vi "Extract Lines on Grass.vi"(8 "error in (no error)":errorcluster, 11 "Image Src":T1) -> (0 "error out":errorcluster, 2 "Number of Particles":i32, 3 "Image Out":T1, 7 "Number of Particles1":i32)   [LabVIEW 2009]
doc: "VI which takes an image and outputs marked regions. One for the left and one for the right"
uses:
  <vilib>/vision/Image Controls.llb/IMAQ Image.ctl
  <vilib>/vision/NI_Vision_Development_Module.lvlib
panel:
  out "Image Dst Out":T1(plugin-control)
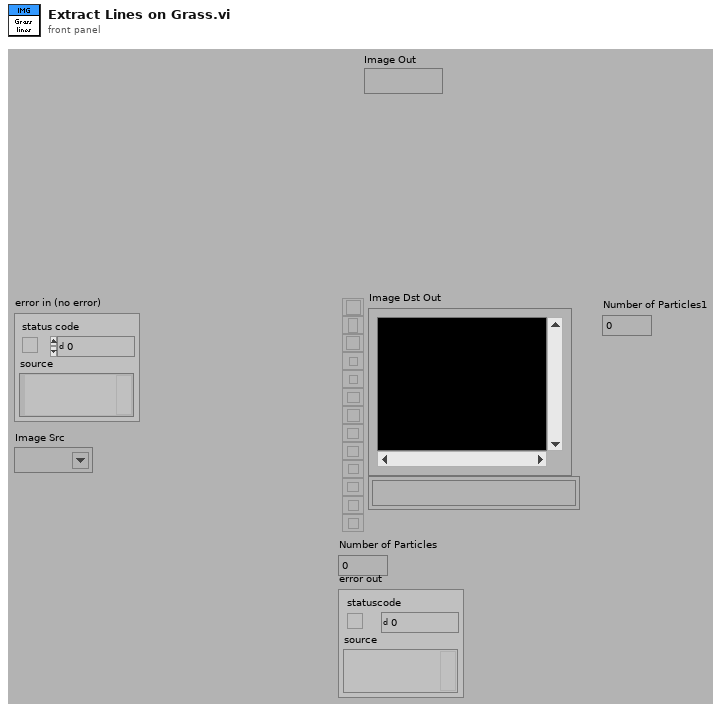
[diagram p1: front panel]
types:
  T1 = typedef "IMAQ Image.ctl" = refnum<image>
  T2 = typedef "Image Type" = u32
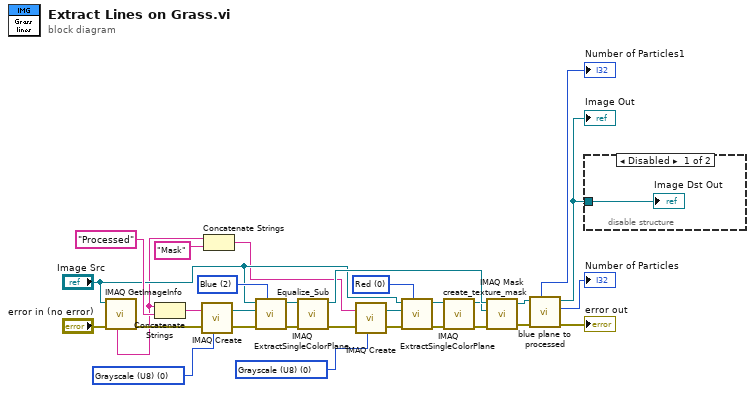
[diagram p0: block diagram]
diagram:
  w18 = T2 0 items=["Grayscale (U8)", "Grayscale (I16)", "Grayscale (SGL)", "Complex (CSG)", "RGB (U32)", "HSL (U32)", "RGB (U64)"] ("Image Type")
  w21 = 0 items=["Red", "Green", "Blue", "Hue", "Saturation", "Luminance", "Value", "Intensity"] ("Color Plane")
  w25 = 2 items=["Red", "Green", "Blue", "Hue", "Saturation", "Luminance", "Value", "Intensity"] ("Color Plane")
  w28 = T2 0 items=["Grayscale (U8)", "Grayscale (I16)", "Grayscale (SGL)", "Complex (CSG)", "RGB (U32)", "HSL (U32)", "RGB (U64)"] ("Image Type")
  n1 = call "IMAQ GetImageInfo"("error in (no error)"="error in (no error)", "Image"="Image Src") -> ("error out"=w10:errorcluster, "Image Name"=w4:string)  [unwired: 8 out]
  n2 = Concatenate Strings(w4, "Processed" ("Image Name")) -> (w6:string)
  n3 = call "IMAQ Create"("Image Name"=w6, "Image Type"=w18, "error in (no error)"=w10) -> ("New Image"=w20:T1, "error out"=w19:errorcluster)  [unwired: 1 in, 1 out]
  n4 = Concatenate Strings(w4, "Mask" ("Image Name")) -> (w7:string)
  n5 = call "IMAQ ExtractSingleColorPlane"("Color Plane"=w25, "error in (no error)"=w19, "Image Dst"=w20, "Image Src"="Image Src") -> ("error out"=w24:errorcluster, "Image Dst Out"=w23:T1)  [unwired: 6 out]
  n6 = call "Equalize_Sub.vi"("error in (no error)"=w24, "Image Src"=w23) -> ("error out"=w27:errorcluster, "Image Out"=w30:T1)  [unwired: 8 out]
  n7 = call "IMAQ Create"("Image Name"=w7, "Image Type"=w28, "error in (no error)"=w27) -> ("New Image"=w17:T1, "error out"=w22:errorcluster)  [unwired: 1 in, 1 out]
  n8 = call "IMAQ ExtractSingleColorPlane"("Color Plane"=w21, "error in (no error)"=w22, "Image Dst"=w17, "Image Src"="Image Src") -> ("error out"=w16:errorcluster, "Image Dst Out"=w12:T1)  [unwired: 6 out]
  n9 = call "create_texture_mask.vi"("error in (no error)"=w16, "Image Src"=w12) -> ("error out"=w29:errorcluster, "Image"=w26:T1)  [unwired: 8 out]
  n10 = call "IMAQ Mask"("error in (no error)"=w29, "Image Mask"=w26, "Image Src"=w30) -> ("error out"=w14:errorcluster, "Image Dst Out"=w15:T1)  [unwired: 1 in, 1 out]
  n11 = call "blue plane to processed.vi"("error in (no error)"=w14, "Image Src"=w15) -> ("error out"=→"error out":errorcluster, "Number of Particles"=→"Number of Particles":i32, "Image Dst Out"=w1:T1, "Number of Particles1"=→"Number of Particles1":i32)  [unwired: 6 out]
  "Image Out" <- w1
  n12 = disable-structure shown="Disabled" {
    disable-tunnel: w1 -> [w31 _]
    frame #0 {
      "Image Dst Out" <- w31
    }
    frame #1 {
    }
  }
